vi "Configure Modulation (IQ).vi"(0 "VISA resource name":refnum<visa-resource-name>, 1 "Enable I/Q Modulator (T:Enable)":bool=TRUE, 2 "Enable Burst Envelop (F:Disable)":bool, 5 "I/Q Source No. (1)":u16(ring)=1 items=["1"=1, "2"=2], 7 "I/Q Source (0: Ext 50 Ohms)":u16(ring) items=["Ext 50 Ohms", "Ext 600 Ohms", "Internal", "Baseband Generator", "Off", "Sum"], 9 "I/Q Signal Source (0: Ext 50 Ohms)":u16(ring) items=["Ext 50 Ohms"=0, "Ext 600 Ohms"=1, "Baseband Generator"=3, "Off"=4], 11 "error in (no error)":errorcluster, 12 "I/Q Phase Polarity (0: Normal)":u16(ring) items=["Normal", "Inverted"], 13 "Summing Ratio (0 dB)":dbl, 14 "Enable High Crest Mode (F:Disable)":bool) -> (4 "VISA resource name out":refnum<visa-resource-name>, 15 "error out":errorcluster)   [LabVIEW 2011, in "Agilent PSG MXG Series.lvlib"]
doc: "Configures the I/Q modulator.\n\n<B>Notes:</B>\n(1) This VI is valid only in E8267C, E8267D, N5182A.\n\n(2) For E8267C, this VI is valid only when the instrument installs <B>Option 002</B> (Internal baseband generator) or <B>Option 602</B> (Digital bus baseband generator)."
uses:
  Agilent PSG MXG Series.lvlib
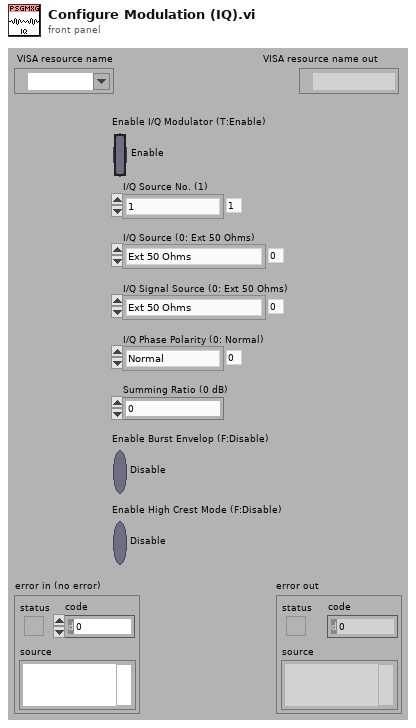
[diagram p1: front panel]
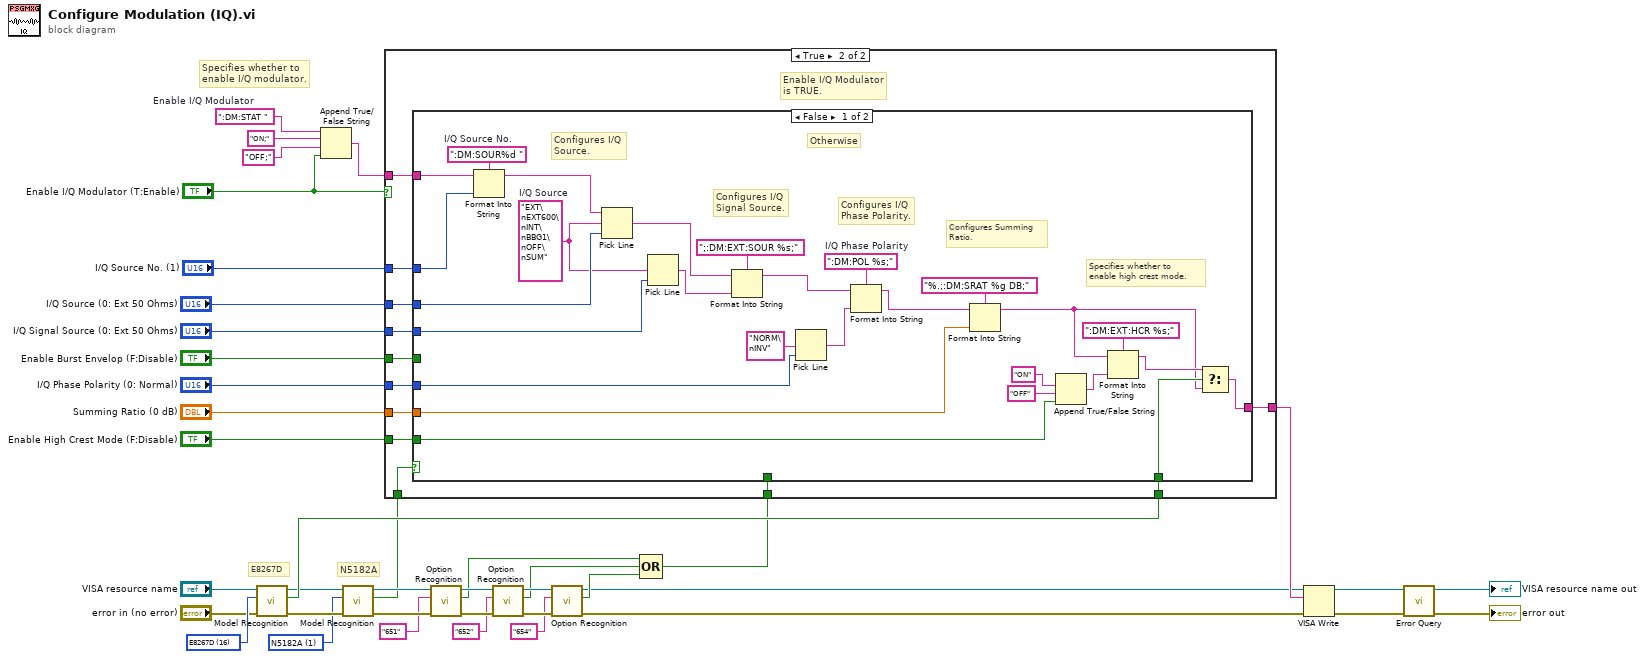
[diagram p0: block diagram]
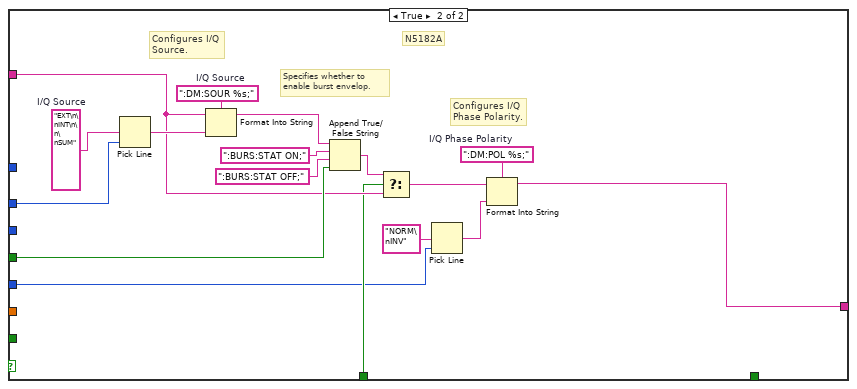
[diagram p3: hidden frame]
diagram:
  w21 = u16 1 items=["N5181A"=0, "N5182A"=1, "E8241A"=5, "E8244A"=6, "E8251A"=7, "E8254A"=8, "E8247C"=10, "E8257C"=11, "E8267C"=12, "E8257D"=15, "E8267D"=16] ("Model Type (0: N5181A)")
  w25 = u16 16 items=["N5181A"=0, "N5182A"=1, "E8241A"=5, "E8244A"=6, "E8251A"=7, "E8254A"=8, "E8247C"=10, "E8257C"=11, "E8267C"=12, "E8257D"=15, "E8267D"=16] ("Model Type (0: N5181A)")
  w40 = ":DM:STAT "  # Enable I/Q Modulator
  # "Specifies whether to\nenable I/Q modulator."
  # "E8267D"
  # "N5182A"
  n1 = call "Model Recognition.vi"("error in (no error)"="error in (no error)", "Model Type (0: N5181A)"=w25, "VISA resource name"="VISA resource name") -> ("error out"=w22:errorcluster, "Is Model Correct"=w24:bool, "VISA resource name out"=w23:refnum<visa-resource-name>)  [unwired: 6 in]
  n2 = Append True/False String(1:"Enable I/Q Modulator (T:Enable)", 2:"OFF;" ("false string"), 3:"ON;" ("true string"), 4:w40) -> (0:w35:string)
  n3 = call "Model Recognition.vi"("error in (no error)"=w22, "Model Type (0: N5181A)"=w21, "VISA resource name"=w23) -> ("error out"=w15:errorcluster, "Is Model Correct"=w4:bool, "VISA resource name out"=w16:refnum<visa-resource-name>)  [unwired: 6 in]
  n4 = call "Option Recognition.vi"("error in (no error)"=w15, "Option (\"\")"="651" ("Option (\"\")"), "VISA resource name"=w16) -> ("error out"=w12:errorcluster, "Is Option Installed"=w7:bool, "VISA resource name out"=w13:refnum<visa-resource-name>)  [unwired: 6 in]
  n5 = call "Option Recognition.vi"("error in (no error)"=w12, "Option (\"\")"="652" ("Option (\"\")"), "VISA resource name"=w13) -> ("error out"=w9:errorcluster, "Is Option Installed"=w6:bool, "VISA resource name out"=w10:refnum<visa-resource-name>)  [unwired: 6 in]
  n6 = call "Option Recognition.vi"("error in (no error)"=w9, "Option (\"\")"="654" ("Option (\"\")"), "VISA resource name"=w10) -> ("error out"=w1:errorcluster, "Is Option Installed"=w5:bool, "VISA resource name out"=w2:refnum<visa-resource-name>)  [unwired: 6 in]
  n7 = Compound Arithmetic op=OR(w7, w6, w5) -> (w3:bool)
  n8 = case shown="True" "Enable I/Q Modulator (T:Enable)" {
    tunnel: "I/Q Source No. (1)" -> [_ w51]
    tunnel: w4 -> [_ w53]
    tunnel: w35 -> [w41 w52]
    tunnel: "I/Q Source (0: Ext 50 Ohms)" -> [_ w50]
    tunnel: "I/Q Signal Source (0: Ext 50 Ohms)" -> [_ w49]
    tunnel: "Enable Burst Envelop (F:Disable)" -> [_ w47]
    tunnel: "I/Q Phase Polarity (0: Normal)" -> [_ w46]
    tunnel: "Summing Ratio (0 dB)" -> [_ w45]
    tunnel: "Enable High Crest Mode (F:Disable)" -> [_ w42]
    tunnel: w24 -> [_ w44]
    tunnel: [w41 w43] -> w26
    tunnel: w3 -> [_ w48]
    frame False {
      # "Enable I/Q Modulator\nis FALSE."
    }
    frame True {
      # "Enable I/Q Modulator\nis TRUE."
      n9 = case shown="False" w53 {
        tunnel: w52 -> [w80 w88]
        tunnel: w51 -> [w79 _]
        tunnel: w50 -> [w77 w96]
        tunnel: w49 -> [w73 _]
        tunnel: w48 -> [_ w87]
        tunnel: w47 -> [_ w90]
        tunnel: w46 -> [w66 w82]
        tunnel: w45 -> [w63 _]
        tunnel: w44 -> [w58 _]
        tunnel: [w55 w81] -> w43
        tunnel: w42 -> [w54 _]
        frame False {
          w70 = ":DM:POL %s;"  # I/Q Phase Polarity
          w74 = "EXT\nEXT600\nINT\nBBG1\nOFF\nSUM"  # I/Q Source
          w76 = ":DM:SOUR%d "  # I/Q Source No.
          # "Specifies whether to\nenable high crest mode."
          # "Configures Summing\nRatio."
          # "Configures I/Q\nPhase Polarity."
          # "Configures I/Q\nSignal Source."
          # "Configures I/Q\nSource."
          # "Otherwise"
          n10 = Format Into String(format string=w76, initial string=w80, w79) -> (resulting string=w78:string)  [unwired: 1 in, 1 out]
          n11 = Pick Line(string ("")=w78, multi-line string=w74, line index=w77) -> (output string=w72:string)
          n12 = Pick Line(multi-line string=w74, line index=w73) -> (output string=w71:string)  [unwired: 1 in]
          n13 = Format Into String(format string=";:DM:EXT:SOUR %s;", initial string=w72, w71) -> (resulting string=w67:string)  [unwired: 1 in, 1 out]
          n14 = Pick Line(multi-line string="NORM\nINV", line index=w66) -> (output string=w69:string)  [unwired: 1 in]
          n15 = Format Into String(format string=w70, initial string=w67, w69) -> (resulting string=w64:string)  [unwired: 1 in, 1 out]
          n16 = Format Into String(format string="%.;:DM:SRAT %g DB;", initial string=w64, w63) -> (resulting string=w56:string)  [unwired: 1 in, 1 out]
          n17 = Append True/False String(1:w54, 2:"OFF" ("false string"), 3:"ON" ("true string")) -> (0:w61:string)  [unwired: 1 in]
          n18 = Format Into String(format string=":DM:EXT:HCR %s;", initial string=w56, w61) -> (resulting string=w57:string)  [unwired: 1 in, 1 out]
          n19 = Select(t=w57, s=w58, f=w56) -> (s? t:f=w55:string)
        }
        frame True {
          w86 = ":DM:POL %s;"  # I/Q Phase Polarity
          w94 = ":DM:SOUR %s;"  # I/Q Source
          w97 = "EXT\n\nINT\n\n\nSUM"  # I/Q Source
          # "Configures I/Q\nPhase Polarity."
          # "Specifies whether to\nenable burst envelop."
          # "Configures I/Q\nSource."
          # "N5182A"
          n20 = Pick Line(multi-line string=w97, line index=w96) -> (output string=w95:string)  [unwired: 1 in]
          n21 = Format Into String(format string=w94, initial string=w88, w95) -> (resulting string=w91:string)  [unwired: 1 in, 1 out]
          n22 = Append True/False String(1:w90, 2:":BURS:STAT OFF;" ("true string"), 3:":BURS:STAT ON;" ("true string"), 4:w91) -> (0:w89:string)
          n23 = Select(t=w89, s=w87, f=w88) -> (s? t:f=w85:string)
          n24 = Pick Line(multi-line string="NORM\nINV", line index=w82) -> (output string=w84:string)  [unwired: 1 in]
          n25 = Format Into String(format string=w86, initial string=w85, w84) -> (resulting string=w81:string)  [unwired: 1 in, 1 out]
        }
      }
    }
  }
  n26 = VISA Write(VISA resource name=w2, write buffer=w26, error in (no error)=w1) -> (VISA resource name out=w29:refnum<visa-resource-name>, error out=w28:errorcluster)  [unwired: 1 out]
  n27 = call "Error Query.vi"("error in (no error)"=w28, "VISA resource name"=w29) -> ("error out"=→"error out":errorcluster, "VISA resource name out"=→"VISA resource name out":refnum<visa-resource-name>)  [unwired: 6 in, 2 out]
